vi "Insert into Subpanel.vi"(8 "error in (no error)":errorcluster, 10 "SubPanel":refnum<vi>, 11 "Express VI Type in":refnum<class "Express VI Type.lvclass">) -> (0 "error out":errorcluster, 3 "Express VI Type out":refnum<class "Express VI Type.lvclass">)   [LabVIEW 2020, in "Peek Window.lvlib" / "Express VI Type.lvclass"]
uses:
  Express VI Type.lvclass
  Express VI Type.lvclass/Express VI Type.ctl
  Implementation VI Type/Implementation VI Type.lvclass
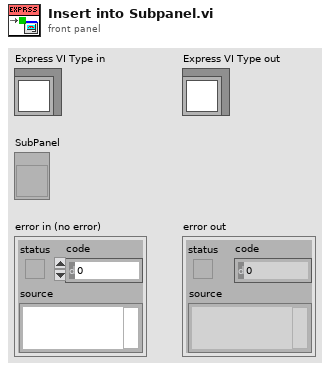
[diagram p1: front panel]
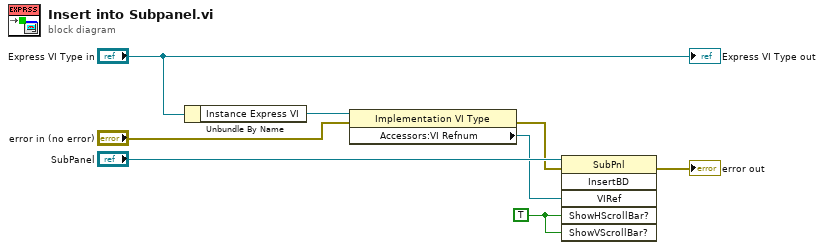
[diagram p0: block diagram]
diagram:
  w8 = TRUE ("ShowHScrollBar")
  n1 = Unbundle By Name("Express VI Type in") -> ("Instance Express VI"=w4:refnum<class "Implementation VI Type.lvclass">)
  n2 = property class="Implementation VI Type"(reference=w4, error in="error in (no error)") -> (error out=w1:errorcluster, "Accessors:VI Refnum"=w3:refnum<vi>)  [unwired: 1 out]
  n3 = invoke on="Invoke Node" class="SubPnl" method="InsertBD"(reference="SubPanel", error in=w1, "VIRef"=w3, "ShowHScrollBar?"=w8, "ShowVScrollBar?"=w8) -> (error out=→"error out":errorcluster)  [unwired: 1 in, 5 out]
  "Express VI Type out" <- "Express VI Type in"
